vi "drawLines.vi"(0 "reference":refnum<class "Graphics.lvclass">, 1 "points":T2[](array[typedef]) {"y" format="%.2f"; "x" format="%.2f"}, 2 "lineWidth(1)":dbl=1.0 format="%.2f", 3 "color(if not used=default color)":u32=536870912 format="%.0x", 4 "fill?(F)":bool, 5 "error in (no error)":errorcluster, 7 "stroke":T1) -> (14 "reference out":refnum<class "Graphics.lvclass">, 19 "error out":errorcluster)   [LabVIEW 2012, in "Graphics.lvclass"]
doc: "Draws lines\nIf point=(NaN,???), The pen will be lifted\nand start over from the next point (put down)."
uses:
  <resource>/Framework/Providers/Open_GDS/UML/Graphics_class/Graphics.lvclass
  <resource>/Framework/Providers/Open_GDS/UML/General/Point/Point Point2D.ctl
  <resource>/Framework/Providers/Open_GDS/UML/Graphics_class/StrokeType.ctl
panel:
  # "Always set\nVI Server class\nto current VI. Do not\nconnect this control\nto the connector pane.\n(Tip!: Just drag\nand drop the icon\ninto the refnum)"
  # "If point=(NaN,???), The pen will be lifted\nand start over from the next point (put down)."
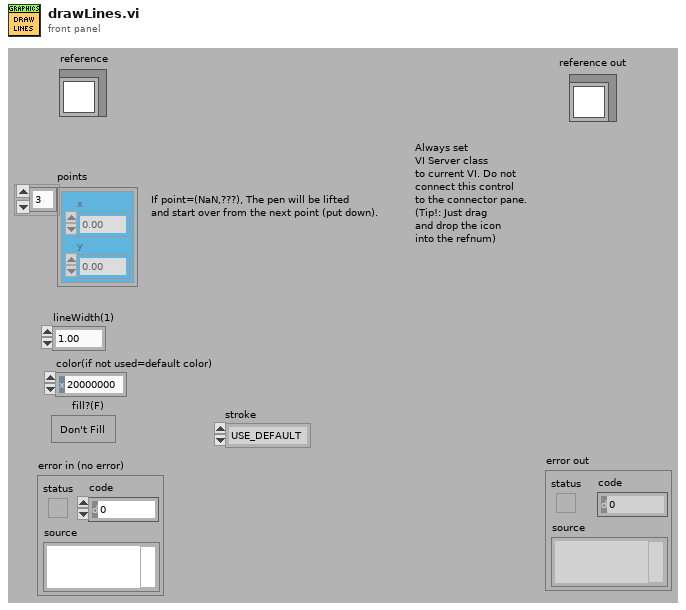
[diagram p1: front panel]
types:
  T1 = typedef "Graphics.lvclass/StrokeType.ctl" = enum16{"USE_DEFAULT", "SOLID", "DOTTED"}
  T2 = typedef "Point Point2D.ctl" = cluster{"x":dbl, "y":dbl}
  T3 = typedef "Graphics.lvclass/ObjectAttributes.ctl" = cluster{"drawColor":u32, "backgroundColor":u32, "font":T4, "fontType":T5, "picture":picture, "stroke":T1, "scaleX":dbl, "scaleY":dbl, "screenRef":refnum<vi>, "offsetX":dbl, "offsetY":dbl}
  T4 = typedef "Graphics.lvclass/FontType.ctl" = cluster{"Font Name:":string, "Size":i16, "Strikeout?":bool, "Italic?":bool, "Underline?":bool, "Outline?":bool, "Shadow?":bool, "Bold?":bool}
  T5 = typedef "Graphics.lvclass/LvFontType.ctl" = enum16{"User-specified Font", "Application Font", "System Font", "Dialog Font"}
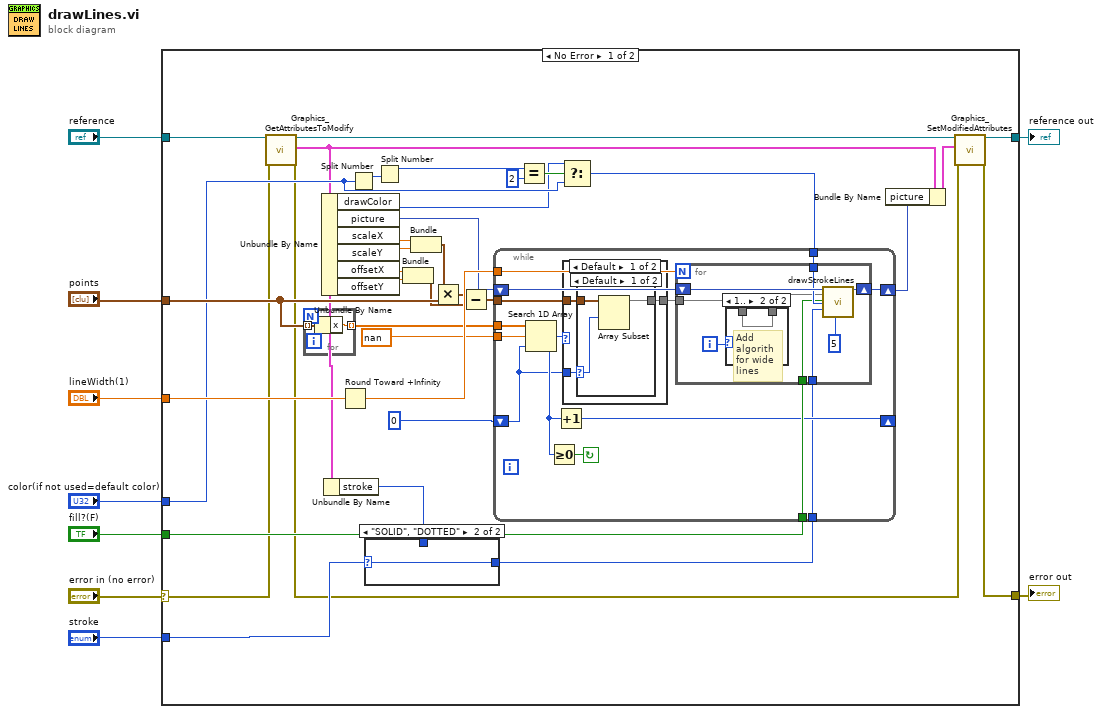
[diagram p0: block diagram]
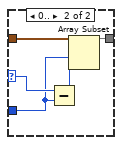
[diagram p4: hidden frame]
diagram:
  n1 = case shown="No Error" "error in (no error)" {
    selector: "error in (no error)" -> [w10 w86]
    tunnel: "reference" -> [w44 w87]
    tunnel: [w43 w86] -> w8
    tunnel: [w42 w87] -> w7
    tunnel: "points" -> [w41 _]
    tunnel: "lineWidth(1)" -> [w40 _]
    tunnel: "color(if not used=default color)" -> [w39 _]
    tunnel: "fill?(F)" -> [w38 _]
    tunnel: "stroke" -> [w37 _]
    frame No Error {
      n2 = call <resource>:"Graphics_GetAttributesToModify.vi"("reference in"=w44, "error in (no error)"=w10) -> ("reference out"=w36:refnum<class "Graphics.lvclass">, "Attributes"=w34:T3, "error out"=w35:errorcluster)  [unwired: 1 in, 14 out]
      n3 = for {
        tunnel: w41 -> [w48] mode=indexing
        tunnel: [w47] -> w21 mode=indexing
        n4 = Unbundle By Name(w48) -> ("x"=w47:dbl)
      }
      n5 = Unbundle By Name(w34) -> ("drawColor"=w27:u32, "picture"=w25:picture, "scaleX"=w19:dbl, "scaleY"=w20:dbl, "offsetX"=w14:dbl, "offsetY"=w15:dbl)
      n6 = Unbundle By Name(w34) -> ("stroke"=w16:T1)
      n7 = Round Toward +Infinity(x=w40) -> (ceil(x): smallest int >= x=w32:dbl)
      n8 = Split Number(x=w39) -> (hi(x)=w31:u16)  [unwired: 1 out]
      n9 = case shown="\"SOLID\", \"DOTTED\"" w37 {
        selector: w37 -> [_ w46]
        tunnel: [w45 w46] -> w17
        tunnel: w16 -> [w45 _]
        frame "USE_DEFAULT", Default {
        }
        frame "SOLID", "DOTTED" {
        }
      }
      n10 = Split Number(x=w31) -> (hi(x)=w30:u8)  [unwired: 1 out]
      n11 = Bundle("offsetX"=w14, "offsetY"=w15) -> (w12:cluster{"offsetX":dbl, "offsetY":dbl})  [unwired: 1 out]
      n12 = Bundle("scaleX"=w19, "scaleY"=w20) -> (w18:cluster{"scaleX":dbl, "scaleY":dbl})  [unwired: 1 out]
      n13 = Multiply(x=w18, y=w41) -> (x*y=w13:T2[])
      n14 = Subtract(x=w13, y=w12) -> (x-y=w11:T2[])
      n15 = Equal?(x=w30, y=u8 2) -> (x = y?=w28:bool)
      n16 = Select(t=w27, s=w28, f=w39) -> (s? t:f=w26:u32)
      n17 = while {
        tunnel: w11 -> [w51]
        tunnel: w32 -> [w62]
        tunnel: w26 -> [w61]
        tunnel: w38 -> [w60]
        shift-right: [w58] -> w24
        shift-left: w25 -> [w59]
        shift-right: [w57] -> _
        shift-left: 0 -> [w52]
        tunnel: nan -> [w56]
        tunnel: w21 -> [w50]
        tunnel: w17 -> [w49]
        stop <- w53 continue-if-true
        n18 = Search 1D Array(1D array=w50, element=w56, start index (0)=w52) -> (index of element=w54:i32)
        n19 = Greater Or Equal To 0?(x=w54) -> (x >= 0?=w53:bool)
        n20 = Increment(x=w54) -> (x+1=w57:i32)
        n21 = case shown="Default" w54 {
          selector: w54 -> [_ w71]
          tunnel: w51 -> [w64 w74]
          tunnel: [w63 w73] -> w55
          tunnel: w52 -> [w65 w70]
          frame Default {
            n22 = case shown="Default" w65 {
              selector: w65 -> [w66 _]
              tunnel: w64 -> [w68 w69]
              tunnel: [w67 w69] -> w63
              frame Default {
                n23 = Array Subset(array=w68, index=w66) -> (w67:T2[])  [unwired: 1 in]
              }
              frame 0 {
              }
            }
          }
          frame 0.. {
            n24 = Subtract(x=w71, y=w70) -> (x-y=w72:i32)
            n25 = Array Subset(array=w74, index=w70, length=w72) -> (w73:T2[])
          }
        }
        n26 = for {
          N: w62 -> [_]
          tunnel: w55 -> [w81]
          tunnel: w61 -> [w82]
          shift-right: [w77] -> w58
          shift-left: w59 -> [w83]
          tunnel: w60 -> [w78]
          tunnel: w49 -> [w76]
          i -> [w80]
          n27 = case shown="1.." w80 {
            tunnel: [w84 w85] -> w79
            tunnel: w81 -> [w84 w85]
            frame 0, Default {
            }
            frame 1.. {
              # "Add algorith for wide lines"
            }
          }
          n28 = call <resource>:"drawStrokeLines.vi"("picture"=w83, "line endpoints"=w79, "fill?(F)"=w78, "color(black)"=w82, "stroke"=w76, "strokeLength"=5) -> ("new picture"=w77:picture)  [unwired: 2 in, 11 out]
        }
      }
      n29 = Bundle By Name(cluster=w34, "picture"=w24) -> (w33:T3)
      n30 = call <resource>:"Graphics_SetModifiedAttributes.vi"("reference in"=w36, "Attributes"=w33, "error in (no error)"=w35) -> ("reference out"=w42:refnum<class "Graphics.lvclass">, "error out"=w43:errorcluster)  [unwired: 3 in, 12 out]
    }
    frame Error {
    }
  }
  "reference out" <- w7
  "error out" <- w8
